vi "Autonomous Independent.vi"() -> ()   [LabVIEW 2014]
doc: "This VI is called when autonomous begins, and will automatically be terminated when autonomous ends. You can carry out timed or sensor driven robot movement independently without needing to return to the caller."
uses:
  <vilib>/Rock Robotics/WPI/SafetyOutput/WPI_SafetyOutputConfigMenu.ctl
  <vilib>/Rock Robotics/WPI/Joystick/WPI_JoystickGetSetRefNum.vi
  AutoVar.vi
  <vilib>/Rock Robotics/WPI/RobotDrive/WPI_RobotDriveGetSetRefNum.vi
  Global 2.vi
  <vilib>/Rock Robotics/WPI/RobotDrive/WPI_RobotDriveArcadeDrive_Standard(NoSaturation).vi
panel:
  out "Current Movement, for debugging":T1 {"Y Joystick Value" scale=1.0..-1.0; "X Joystick Value" scale=-1.0..1.0}
  in  "Array of robot movements":T2(array[cluster]) {"Y Joystick Value" scale=1.0..-1.0; "X Joystick Value" scale=-1.0..1.0}
  # "Be sure to right-click and choose Data Operations>>Make Current Value default if you want to save the array values with the VI"
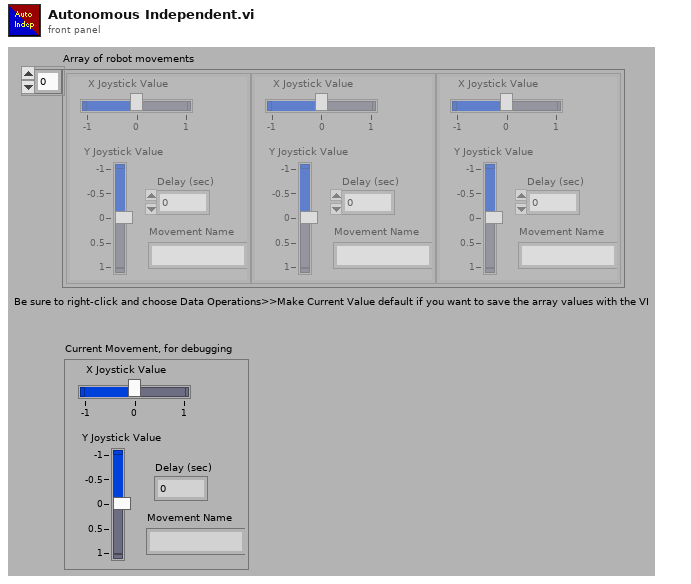
[diagram p1: front panel]
types:
  T1 = cluster{"X Joystick Value":dbl, "Y Joystick Value":dbl, "Delay (sec)":dbl, "Movement Name":string}
  T2 = cluster{"X Joystick Value":dbl, "Y Joystick Value":dbl, "Delay (sec)":dbl, "Movement Name":string}[]
  T3 = typedef "WPI_SafetyOutputConfigMenu.ctl" = enum16{"Enable", "Disable"}
  T4 = typedef "WPI_MotorControlDeviceRef.ctl" = cluster{"DeviceStatus":errorcluster, "Type":T5, "PWM":cluster{"Controller":T6, "PWM Channel":T7, "DeadBand":T8}, "CAN":cluster{"Device Number":u8, "Control Mode":T9, "Semaphore":T10, "Max Vout":dbl, "TalonSRX Control Mode":T11}, "Invert":bool, "TransformRef":T12, "InvTransformRef":T12}
  T5 = typedef "WPI_MotorControlType.ctl" = enum16{"PWM", "CAN", "CANTalonSRX"}
  T6 = typedef "FPGA_TypedefDigitalModule.ctl" = enum16{"Controller 1"}
  T7 = typedef "FPGA_DIOPWMChannel.ctl" = enum8{"PWM 0", "PWM 1", "PWM 2", "PWM 3", "PWM 4", "PWM 5", "PWM 6", "PWM 7", "PWM 8", "PWM 9", "PWM MXP 0", "PWM MXP 1", "PWM MXP 2", "PWM MXP 3", "PWM MXP 4", "PWM MXP 5", "PWM MXP 6", "PWM MXP 7", "PWM MXP 8", "PWM MXP 9", "Invalid"}
  T8 = typedef "WPI_PWMDeadband.ctl" = cluster{"Name":string, "maxPositivePwm":i32, "minPositivePwm":i32, "centerPwm":i32, "maxNegativePwm":i32, "minNegativePwm":i32, "angularRange":u16}
  T9 = typedef "WPI_CANJaguar_ControlMode.ctl" = enum8{"Percent VBus", "Current", "Speed", "Position", "Voltage"}
  T10 = typedef "Semaphore RefNum" = refnum<k1>
  T11 = typedef "WPI_CANTalonSRX_APIControlMode.ctl" = enum8{"Percent VBus", "Speed", "Position", "Slave", "Unchanged / Invalid"}
  T12 = typedef "WPI_PWMTransform_ConPane.ctl" = refnum<vi>
  T13 = typedef "WPI_RobotDriveDevRef.ctl" = cluster{"DevStatus":errorcluster, "Motors[]":T4[], "Square Inputs":bool, "Max Output":dbl}
  T14 = typedef "WPI_JoystickDevRef.ctl" = cluster{"Device":T15}
  T15 = typedef "WPI_JoystickDeviceEnum.ctl" = enum16{"USB 0", "USB 1", "USB 2", "USB 3", "USB 4", "USB 5"}
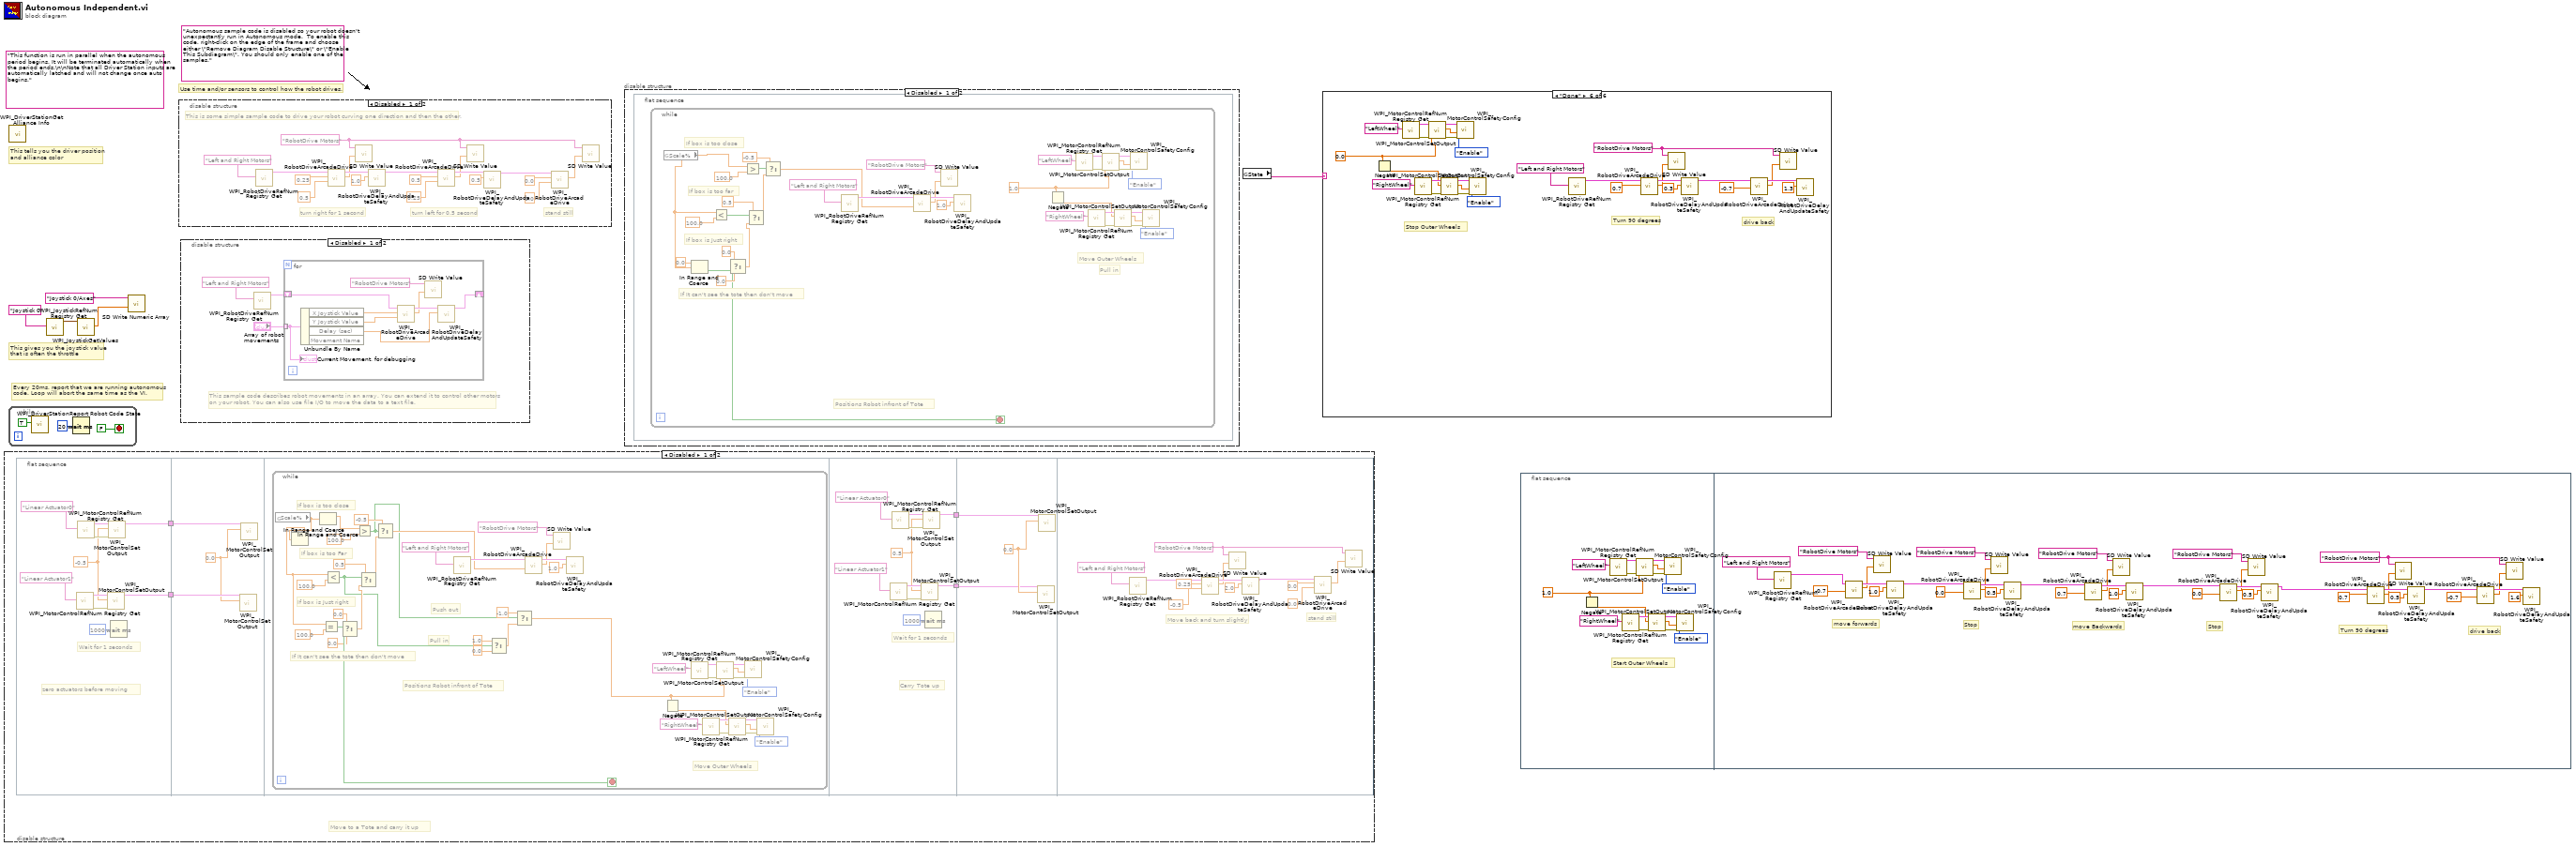
[diagram p0: block diagram]
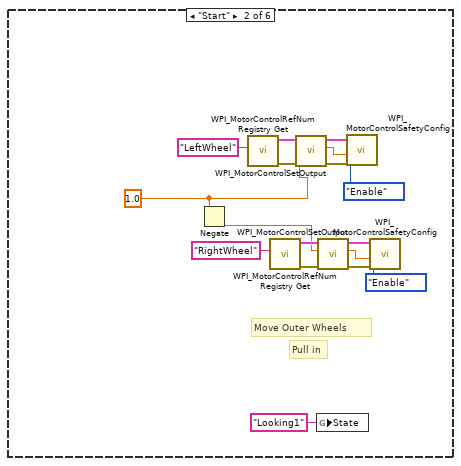
[diagram p4: hidden frame]
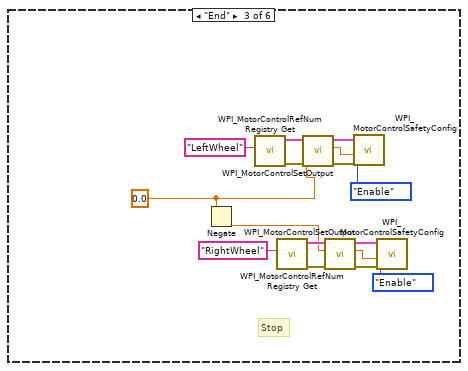
[diagram p5: hidden frame]
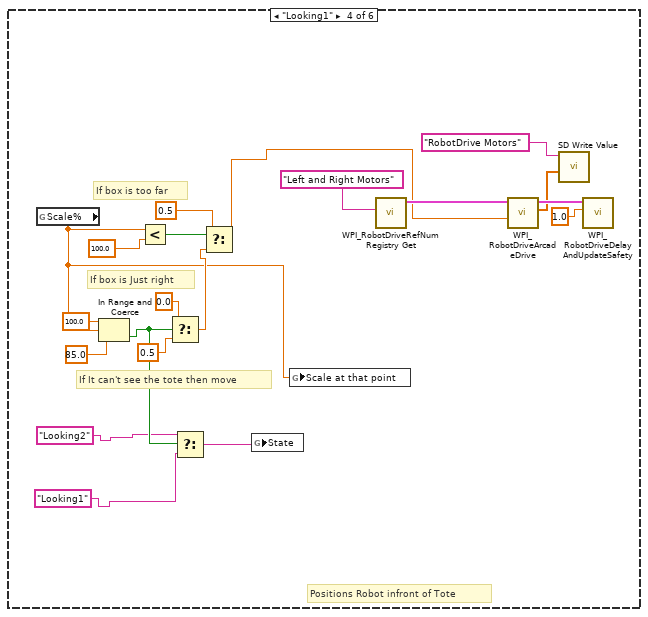
[diagram p6: hidden frame]
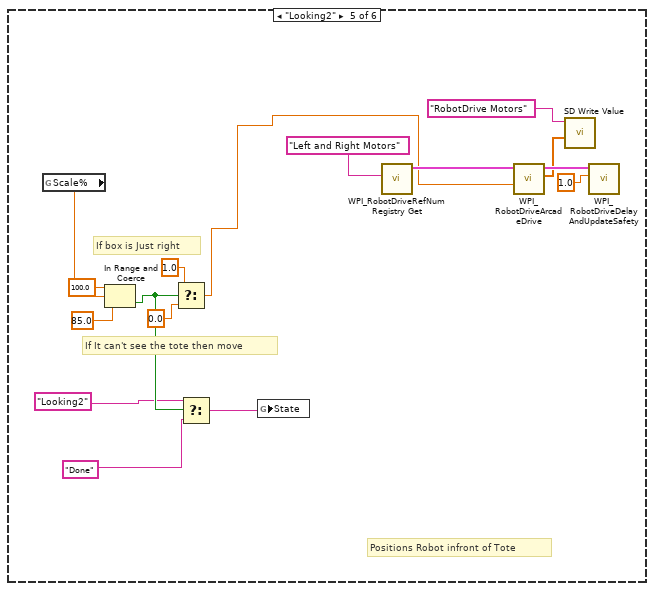
[diagram p7: hidden frame]
diagram:
  (unwired) "Autonomous sample code is disabled so your robot doesn't unexpectantly run in Autonomous mode.  To enable this code, right-click on the edge of the frame and choose either \"Remove Diagram Disable Structure\" or \"Enable This Subdiagram\". You should only enable one of the samples."
  (unwired) "This function is run in parallel when the autonomous period begins. It will be terminated automatically when the period ends.\n\nNote that all Driver Station inputs are automatically latched and will not change once auto begins."
  # "Every 20ms, report that we are running autonomous\ncode. Loop will abort the same time as the VI."
  # "This gives you the joystick value\nthat is often the throttle"
  # "Use time and/or sensors to control how the robot drives."
  # "This tells you the driver position\nand alliance color"
  n1 = disable-structure shown="Disabled" {
    frame Disabled {
      # "Move to a Tote and carry it up"
      n2 = flat-sequence {
        tunnel: [w11] -> w9
        tunnel: [w10] -> w8
        tunnel: w9 -> [w22]
        tunnel: w8 -> [w21]
        tunnel: [w66] -> w7
        tunnel: [w65] -> w6
        tunnel: w7 -> [w76]
        tunnel: w6 -> [w75]
        frame #0 {
          w13 = -0.5 ("Output")
          # "zero actuators before moving"
          # "Wait for 1 seconds"
          n3 = call <vilib>:"WPI_MotorControlRefNum Registry Get.vi"("refnum name"="Linear Actuator1") -> ("error out"=w16:errorcluster, "MotorControlDevRef"=w15:T4)  [unwired: 9 in]
          n4 = call <vilib>:"WPI_MotorControlRefNum Registry Get.vi"("refnum name"="Linear Actuator0") -> ("error out"=w19:errorcluster, "MotorControlDevRef"=w18:T4)  [unwired: 9 in]
          n5 = call <vilib>:"WPI_MotorControlSetOutput.vi"("error in (no error)"=w16, "Output"=w13, "MotorControlDevRef"=w15) -> ("MotorControlDevRef"=w10:T4)  [unwired: 6 in, 2 out]
          n6 = call <vilib>:"WPI_MotorControlSetOutput.vi"("error in (no error)"=w19, "Output"=w13, "MotorControlDevRef"=w18) -> ("MotorControlDevRef"=w11:T4)  [unwired: 6 in, 2 out]
          n7 = Wait (ms)(milliseconds to wait=u32 1000) -> ()  [unwired: 1 out]
        }
        frame #1 {
          w20 = 0.0 ("Output")
          n8 = call <vilib>:"WPI_MotorControlSetOutput.vi"("Output"=w20, "MotorControlDevRef"=w21) -> ()  [unwired: 7 in, 3 out]
          n9 = call <vilib>:"WPI_MotorControlSetOutput.vi"("Output"=w20, "MotorControlDevRef"=w22) -> ()  [unwired: 7 in, 3 out]
        }
        frame #2 {
          n10 = while {
            stop <- w49 stop-if-true
            # "Move Outer Wheels"
            # "Pull in"
            # "Push out"
            # "If It can't see the tote then don't move"
            # "Positions Robot infront of Tote"
            # "If box is Just right"
            # "If box is too Far"
            # "If box is too close"
            n11 = global read "Global 2.vi" "Scale%"() -> (w24:dbl)
            n12 = In Range and Coerce(x=w24) -> (coerced(x)=w23:dbl)  [unwired: 2 in, 1 out]
            n13 = In Range and Coerce(x=w24) -> (coerced(x)=w25:dbl)  [unwired: 2 in, 1 out]
            n14 = Equal?(x=w23, y=100.0) -> (x = y?=w49:bool)
            n15 = Less?(x=w23, y=100.0) -> (x < y?=w28:bool)
            n16 = Select(t=0.0, s=w49, f=0.0) -> (s? t:f=w57:dbl)
            n17 = Greater?(x=w25, y=100.0) -> (0:w33:bool)
            n18 = Select(t=0.5, s=w28, f=w57) -> (s? t:f=w60:dbl)
            n19 = Select(t=-0.5, s=w33, f=w60) -> (s? t:f=w50:dbl)
            n20 = call <vilib>:"WPI_RobotDriveRefNum Registry Get.vi"("refnum name"="Left and Right Motors") -> ("RobotDriveDevRef"=w53:T13)  [unwired: 1 in, 9 out]
            n21 = Select(t=1.0, s=w28, f=0.0) -> (s? t:f=w29:dbl)
            n22 = Select(t=-1.0, s=w33, f=w29) -> (s? t:f=w31:dbl)
            n23 = call-poly <vilib>:"WPI_RobotDriveArcadeDrive.vi"("Y axis value"=w50, "RobotDriveDevRef"=w53) -> ("Motor Values"=w52:dbl[], "RobotDriveDevRef"=w56:T13)  [unwired: 2 in, 6 out]
            n24 = call-poly <vilib>:"SD Write Value.vi"("Numeric Array"=w52, "Name"="RobotDrive Motors") -> ()  [unwired: 8 in, 2 out]
            n25 = call <vilib>:"WPI_RobotDriveDelayAndUpdateSafety.vi"("Delay (s)"=1.0, "RobotDriveDevRef"=w56) -> ()  [unwired: 8 in, 2 out]
            n26 = Negate(x=w31) -> (-x=w30:dbl)
            n27 = call <vilib>:"WPI_MotorControlRefNum Registry Get.vi"("refnum name"="LeftWheel") -> ("error out"=w47:errorcluster, "MotorControlDevRef"=w46:T4)  [unwired: 9 in]
            n28 = call <vilib>:"WPI_MotorControlRefNum Registry Get.vi"("refnum name"="RightWheel") -> ("error out"=w45:errorcluster, "MotorControlDevRef"=w44:T4)  [unwired: 9 in]
            n29 = call <vilib>:"WPI_MotorControlSetOutput.vi"("error in (no error)"=w47, "Output"=w31, "MotorControlDevRef"=w46) -> ("error out"=w41:errorcluster, "Motor Output"=w40:dbl, "MotorControlDevRef"=w39:T4)  [unwired: 6 in]
            n30 = call <vilib>:"WPI_MotorControlSetOutput.vi"("error in (no error)"=w45, "Output"=w30, "MotorControlDevRef"=w44) -> ("error out"=w38:errorcluster, "Motor Output"=w37:dbl, "MotorControlDevRef"=w36:T4)  [unwired: 6 in]
            n31 = call <vilib>:"WPI_MotorControlSafetyConfig.vi"("error in (no error)"=w41, "timeout (s)"=w40, "mode"=WPI_SafetyOutputConfigMenu."Enable", "MotorControlDevRef"=w39) -> ()  [unwired: 6 in, 2 out]
            n32 = call <vilib>:"WPI_MotorControlSafetyConfig.vi"("error in (no error)"=w38, "timeout (s)"=w37, "mode"=WPI_SafetyOutputConfigMenu."Enable", "MotorControlDevRef"=w36) -> ()  [unwired: 6 in, 2 out]
          }
        }
        frame #3 {
          w68 = 0.5 ("Output")
          # "Carry Tote up"
          # "Wait for 1 seconds"
          n33 = call <vilib>:"WPI_MotorControlRefNum Registry Get.vi"("refnum name"="Linear Actuator1") -> ("error out"=w71:errorcluster, "MotorControlDevRef"=w70:T4)  [unwired: 9 in]
          n34 = call <vilib>:"WPI_MotorControlRefNum Registry Get.vi"("refnum name"="Linear Actuator0") -> ("error out"=w74:errorcluster, "MotorControlDevRef"=w73:T4)  [unwired: 9 in]
          n35 = call <vilib>:"WPI_MotorControlSetOutput.vi"("error in (no error)"=w71, "Output"=w68, "MotorControlDevRef"=w70) -> ("MotorControlDevRef"=w65:T4)  [unwired: 6 in, 2 out]
          n36 = call <vilib>:"WPI_MotorControlSetOutput.vi"("error in (no error)"=w74, "Output"=w68, "MotorControlDevRef"=w73) -> ("MotorControlDevRef"=w66:T4)  [unwired: 6 in, 2 out]
          n37 = Wait (ms)(milliseconds to wait=u32 1000) -> ()  [unwired: 1 out]
        }
        frame #4 {
          w77 = 0.0 ("Output")
          n38 = call <vilib>:"WPI_MotorControlSetOutput.vi"("Output"=w77, "MotorControlDevRef"=w75) -> ()  [unwired: 7 in, 3 out]
          n39 = call <vilib>:"WPI_MotorControlSetOutput.vi"("Output"=w77, "MotorControlDevRef"=w76) -> ()  [unwired: 7 in, 3 out]
        }
        frame #5 {
          w78 = "RobotDrive Motors" ("Name")
          # "stand still"
          # "Move back and turn slightly"
          n40 = call <vilib>:"WPI_RobotDriveRefNum Registry Get.vi"("refnum name"="Left and Right Motors") -> ("RobotDriveDevRef"=w85:T13)  [unwired: 1 in, 9 out]
          n41 = call-poly <vilib>:"WPI_RobotDriveArcadeDrive.vi"("Y axis value"=-0.5 ("X axis value"), "X axis value"=0.25, "RobotDriveDevRef"=w85) -> ("Motor Values"=w84:dbl[], "RobotDriveDevRef"=w88:T13)  [unwired: 1 in, 6 out]
          n42 = call-poly <vilib>:"SD Write Value.vi"("Numeric Array"=w84, "Name"=w78) -> ()  [unwired: 8 in, 2 out]
          n43 = call <vilib>:"WPI_RobotDriveDelayAndUpdateSafety.vi"("Delay (s)"=2.0, "RobotDriveDevRef"=w88) -> ("RobotDriveDevRef 2"=w79:T13)  [unwired: 8 in, 1 out]
          n44 = call-poly <vilib>:"WPI_RobotDriveArcadeDrive.vi"("Y axis value"=0.0 ("X axis value"), "X axis value"=0.0, "RobotDriveDevRef"=w79) -> ("Motor Values"=w80:dbl[])  [unwired: 1 in, 7 out]
          n45 = call-poly <vilib>:"SD Write Value.vi"("Numeric Array"=w80, "Name"=w78) -> ()  [unwired: 8 in, 2 out]
        }
      }
    }
    frame Enabled {
    }
  }
  n46 = while {
    stop <- FALSE stop-if-true
    n47 = call <vilib>:"WPI_DriverStationReport Robot Code State.vi"("Autonomous"=TRUE) -> ()  [unwired: 10 in, 1 out]
    n48 = Wait (ms)(milliseconds to wait=u32 20) -> ()  [unwired: 1 out]
  }
  n49 = call <vilib>:"WPI_DriverStationGet Alliance Info.vi"() -> ()  [unwired: 12 out]
  n50 = call <vilib>:"WPI_JoystickRefNum Registry Get.vi"("refnum name"="Joystick 0") -> ("JoystickDevRef"=w4:T14)  [unwired: 1 in, 9 out]
  n51 = call <vilib>:"WPI_JoystickGetValues.vi"("JoystickDevRef"=w4) -> ("Axes"=w2:dbl[])  [unwired: 6 in, 4 out]
  n52 = call <vilib>:"SD Write Numeric Array.vi"("Numeric Array"=w2, "Name"="Joystick 0/Axes") -> ()  [unwired: 8 in, 2 out]
  n53 = disable-structure shown="Disabled" {
    frame Disabled {
      w93 = "RobotDrive Motors" ("Name")
      # "This is some simple sample code to drive your robot curving one direction and then the other."
      # "stand still"
      # "turn left for 0.5 second"
      # "turn right for 1 second"
      n54 = call <vilib>:"WPI_RobotDriveRefNum Registry Get.vi"("refnum name"="Left and Right Motors") -> ("RobotDriveDevRef"=w97:T13)  [unwired: 1 in, 9 out]
      n55 = call-poly <vilib>:"WPI_RobotDriveArcadeDrive.vi"("Y axis value"=0.5 ("X axis value"), "X axis value"=0.25, "RobotDriveDevRef"=w97) -> ("Motor Values"=w96:dbl[], "RobotDriveDevRef"=w104:T13)  [unwired: 1 in, 6 out]
      n56 = call-poly <vilib>:"SD Write Value.vi"("Numeric Array"=w96, "Name"=w93) -> ()  [unwired: 8 in, 2 out]
      n57 = call <vilib>:"WPI_RobotDriveDelayAndUpdateSafety.vi"("Delay (s)"=1.0, "RobotDriveDevRef"=w104) -> ("RobotDriveDevRef 2"=w103:T13)  [unwired: 8 in, 1 out]
      n58 = call-poly <vilib>:"WPI_RobotDriveArcadeDrive.vi"("Y axis value"=0.25 ("X axis value"), "X axis value"=0.5, "RobotDriveDevRef"=w103) -> ("Motor Values"=w95:dbl[], "RobotDriveDevRef"=w102:T13)  [unwired: 1 in, 6 out]
      n59 = call-poly <vilib>:"SD Write Value.vi"("Numeric Array"=w95, "Name"=w93) -> ()  [unwired: 8 in, 2 out]
      n60 = call <vilib>:"WPI_RobotDriveDelayAndUpdateSafety.vi"("Delay (s)"=0.5, "RobotDriveDevRef"=w102) -> ("RobotDriveDevRef 2"=w101:T13)  [unwired: 8 in, 1 out]
      n61 = call-poly <vilib>:"WPI_RobotDriveArcadeDrive.vi"("Y axis value"=0.0 ("X axis value"), "X axis value"=0.0, "RobotDriveDevRef"=w101) -> ("Motor Values"=w94:dbl[])  [unwired: 1 in, 7 out]
      n62 = call-poly <vilib>:"SD Write Value.vi"("Numeric Array"=w94, "Name"=w93) -> ()  [unwired: 8 in, 2 out]
    }
    frame Enabled {
    }
  }
  n63 = disable-structure shown="Disabled" {
    frame Disabled {
      # "This sample code describes robot movements in an array. You can extend it to control other motors\non your robot. You can also use file I/O to move the data to a text file."
      n64 = call <vilib>:"WPI_RobotDriveRefNum Registry Get.vi"("refnum name"="Left and Right Motors") -> ("RobotDriveDevRef"=w112:T13)  [unwired: 1 in, 9 out]
      n65 = for {
        shift-right: [w120] -> _
        shift-left: w112 -> [w121]
        tunnel: "Array of robot movements" -> [w116] mode=indexing
        n66 = Unbundle By Name(w116) -> ("X Joystick Value"=w119:dbl, "Y Joystick Value"=w118:dbl, "Delay (sec)"=w117:dbl)  [unwired: 1 out]
        n67 = call-poly <vilib>:"WPI_RobotDriveArcadeDrive.vi"("Y axis value"=w118, "X axis value"=w119, "RobotDriveDevRef"=w121) -> ("Motor Values"=w114:dbl[], "RobotDriveDevRef"=w122:T13)  [unwired: 1 in, 6 out]
        n68 = call-poly <vilib>:"SD Write Value.vi"("Numeric Array"=w114, "Name"="RobotDrive Motors") -> ()  [unwired: 8 in, 2 out]
        n69 = call <vilib>:"WPI_RobotDriveDelayAndUpdateSafety.vi"("Delay (s)"=w117, "RobotDriveDevRef"=w122) -> ("RobotDriveDevRef 2"=w120:T13)  [unwired: 8 in, 1 out]
        "Current Movement, for debugging" <- w116
      }
    }
    frame Enabled {
    }
  }
  n70 = disable-structure shown="Disabled" {
    frame Disabled {
      n71 = flat-sequence {
        frame #0 {
          n72 = while {
            stop <- w126 stop-if-true
            w123 = 1.0 ("t")
            # "Move Outer Wheels"
            # "Pull in"
            # "If It can't see the tote then don't move"
            # "Positions Robot infront of Tote"
            # "If box is Just right"
            # "If box is too far"
            # "If box is too close"
            n73 = global read "Global 2.vi" "Scale%"() -> (w125:dbl)
            n74 = In Range and Coerce(upper limit=0.0, x=w125) -> (In Range?=w126:bool)  [unwired: 1 in, 1 out]
            n75 = Less?(x=w125, y=100.0) -> (x < y?=w127:bool)
            n76 = Select(t=0.0, s=w126, f=0.0) -> (s? t:f=w152:dbl)
            n77 = Greater?(x=w125, y=100.0) -> (0:w129:bool)
            n78 = Select(t=0.5, s=w127, f=w152) -> (s? t:f=w154:dbl)
            n79 = Select(t=-0.5, s=w129, f=w154) -> (s? t:f=w145:dbl)
            n80 = call <vilib>:"WPI_RobotDriveRefNum Registry Get.vi"("refnum name"="Left and Right Motors") -> ("RobotDriveDevRef"=w148:T13)  [unwired: 1 in, 9 out]
            n81 = call-poly <vilib>:"WPI_RobotDriveArcadeDrive.vi"("Y axis value"=w145, "RobotDriveDevRef"=w148) -> ("Motor Values"=w147:dbl[], "RobotDriveDevRef"=w151:T13)  [unwired: 2 in, 6 out]
            n82 = call-poly <vilib>:"SD Write Value.vi"("Numeric Array"=w147, "Name"="RobotDrive Motors") -> ()  [unwired: 8 in, 2 out]
            n83 = call <vilib>:"WPI_RobotDriveDelayAndUpdateSafety.vi"("Delay (s)"=1.0, "RobotDriveDevRef"=w151) -> ()  [unwired: 8 in, 2 out]
            n84 = Negate(x=w123) -> (-x=w128:dbl)
            n85 = call <vilib>:"WPI_MotorControlRefNum Registry Get.vi"("refnum name"="LeftWheel") -> ("error out"=w143:errorcluster, "MotorControlDevRef"=w142:T4)  [unwired: 9 in]
            n86 = call <vilib>:"WPI_MotorControlRefNum Registry Get.vi"("refnum name"="RightWheel") -> ("error out"=w141:errorcluster, "MotorControlDevRef"=w140:T4)  [unwired: 9 in]
            n87 = call <vilib>:"WPI_MotorControlSetOutput.vi"("error in (no error)"=w143, "Output"=w123, "MotorControlDevRef"=w142) -> ("error out"=w137:errorcluster, "Motor Output"=w136:dbl, "MotorControlDevRef"=w135:T4)  [unwired: 6 in]
            n88 = call <vilib>:"WPI_MotorControlSetOutput.vi"("error in (no error)"=w141, "Output"=w128, "MotorControlDevRef"=w140) -> ("error out"=w134:errorcluster, "Motor Output"=w133:dbl, "MotorControlDevRef"=w132:T4)  [unwired: 6 in]
            n89 = call <vilib>:"WPI_MotorControlSafetyConfig.vi"("error in (no error)"=w137, "timeout (s)"=w136, "mode"=WPI_SafetyOutputConfigMenu."Enable", "MotorControlDevRef"=w135) -> ()  [unwired: 6 in, 2 out]
            n90 = call <vilib>:"WPI_MotorControlSafetyConfig.vi"("error in (no error)"=w134, "timeout (s)"=w133, "mode"=WPI_SafetyOutputConfigMenu."Enable", "MotorControlDevRef"=w132) -> ()  [unwired: 6 in, 2 out]
          }
        }
      }
    }
    frame Enabled {
    }
  }
  n91 = global read "AutoVar.vi" "State"() -> (w1:string)
  n92 = case shown="\"Done\"" w1 {
    frame "False", Default {
    }
    frame "Start" {
      w160 = 1.0 ("t")
      # "Move Outer Wheels"
      # "Pull in"
      n93 = Negate(x=w160) -> (-x=w161:dbl)
      n94 = call <vilib>:"WPI_MotorControlRefNum Registry Get.vi"("refnum name"="LeftWheel") -> ("error out"=w175:errorcluster, "MotorControlDevRef"=w174:T4)  [unwired: 9 in]
      n95 = call <vilib>:"WPI_MotorControlRefNum Registry Get.vi"("refnum name"="RightWheel") -> ("error out"=w173:errorcluster, "MotorControlDevRef"=w172:T4)  [unwired: 9 in]
      n96 = call <vilib>:"WPI_MotorControlSetOutput.vi"("error in (no error)"=w175, "Output"=w160, "MotorControlDevRef"=w174) -> ("error out"=w169:errorcluster, "Motor Output"=w168:dbl, "MotorControlDevRef"=w167:T4)  [unwired: 6 in]
      n97 = global write "AutoVar.vi" "State"("Looking1" ("State")) -> ()
      n98 = call <vilib>:"WPI_MotorControlSetOutput.vi"("error in (no error)"=w173, "Output"=w161, "MotorControlDevRef"=w172) -> ("error out"=w166:errorcluster, "Motor Output"=w165:dbl, "MotorControlDevRef"=w164:T4)  [unwired: 6 in]
      n99 = call <vilib>:"WPI_MotorControlSafetyConfig.vi"("error in (no error)"=w169, "timeout (s)"=w168, "mode"=WPI_SafetyOutputConfigMenu."Enable", "MotorControlDevRef"=w167) -> ()  [unwired: 6 in, 2 out]
      n100 = call <vilib>:"WPI_MotorControlSafetyConfig.vi"("error in (no error)"=w166, "timeout (s)"=w165, "mode"=WPI_SafetyOutputConfigMenu."Enable", "MotorControlDevRef"=w164) -> ()  [unwired: 6 in, 2 out]
    }
    frame "End" {
      w176 = 0.0 ("t")
      # "Stop"
      n101 = Negate(x=w176) -> (-x=w177:dbl)
      n102 = call <vilib>:"WPI_MotorControlRefNum Registry Get.vi"("refnum name"="LeftWheel") -> ("error out"=w191:errorcluster, "MotorControlDevRef"=w190:T4)  [unwired: 9 in]
      n103 = call <vilib>:"WPI_MotorControlRefNum Registry Get.vi"("refnum name"="RightWheel") -> ("error out"=w189:errorcluster, "MotorControlDevRef"=w188:T4)  [unwired: 9 in]
      n104 = call <vilib>:"WPI_MotorControlSetOutput.vi"("error in (no error)"=w191, "Output"=w176, "MotorControlDevRef"=w190) -> ("error out"=w185:errorcluster, "Motor Output"=w184:dbl, "MotorControlDevRef"=w183:T4)  [unwired: 6 in]
      n105 = call <vilib>:"WPI_MotorControlSetOutput.vi"("error in (no error)"=w189, "Output"=w177, "MotorControlDevRef"=w188) -> ("error out"=w182:errorcluster, "Motor Output"=w181:dbl, "MotorControlDevRef"=w180:T4)  [unwired: 6 in]
      n106 = call <vilib>:"WPI_MotorControlSafetyConfig.vi"("error in (no error)"=w185, "timeout (s)"=w184, "mode"=WPI_SafetyOutputConfigMenu."Enable", "MotorControlDevRef"=w183) -> ()  [unwired: 6 in, 2 out]
      n107 = call <vilib>:"WPI_MotorControlSafetyConfig.vi"("error in (no error)"=w182, "timeout (s)"=w181, "mode"=WPI_SafetyOutputConfigMenu."Enable", "MotorControlDevRef"=w180) -> ()  [unwired: 6 in, 2 out]
    }
    frame "Looking1" {
      # "If It can't see the tote then move"
      # "Positions Robot infront of Tote"
      # "If box is Just right"
      # "If box is too far"
      n108 = global read "Global 2.vi" "Scale%"() -> (w194:dbl)
      n109 = In Range and Coerce(upper limit=100.0, x=w194, lower limit=85.0) -> (In Range?=w196:bool)  [unwired: 1 out]
      n110 = Less?(x=w194, y=100.0) -> (x < y?=w201:bool)
      n111 = Select(t=0.0, s=w196, f=0.5) -> (s? t:f=w208:dbl)
      n112 = Select(t="Looking2", s=w196, f="Looking1" ("t")) -> (s? t:f=w195:string)
      n113 = Select(t=0.5, s=w201, f=w208) -> (s? t:f=w198:dbl)
      n114 = global write "AutoVar.vi" "State"(w195) -> ()
      n115 = global write "AutoVar.vi" "Scale at that point"(w194) -> ()
      n116 = call <vilib>:"WPI_RobotDriveRefNum Registry Get.vi"("refnum name"="Left and Right Motors") -> ("RobotDriveDevRef"=w204:T13)  [unwired: 1 in, 9 out]
      n117 = call-poly <vilib>:"WPI_RobotDriveArcadeDrive.vi"("Y axis value"=w198, "RobotDriveDevRef"=w204) -> ("Motor Values"=w203:dbl[], "RobotDriveDevRef"=w207:T13)  [unwired: 2 in, 6 out]
      n118 = call-poly <vilib>:"SD Write Value.vi"("Numeric Array"=w203, "Name"="RobotDrive Motors") -> ()  [unwired: 8 in, 2 out]
      n119 = call <vilib>:"WPI_RobotDriveDelayAndUpdateSafety.vi"("Delay (s)"=1.0, "RobotDriveDevRef"=w207) -> ()  [unwired: 8 in, 2 out]
    }
    frame "Looking2" {
      # "If It can't see the tote then move"
      # "Positions Robot infront of Tote"
      # "If box is Just right"
      n120 = global read "Global 2.vi" "Scale%"() -> (w220:dbl)
      n121 = In Range and Coerce(upper limit=100.0, x=w220, lower limit=85.0) -> (In Range?=w216:bool)  [unwired: 1 out]
      n122 = Select(t=1.0, s=w216, f=0.0) -> (s? t:f=w214:dbl)
      n123 = Select(t="Looking2", s=w216, f="Done" ("t")) -> (s? t:f=w215:string)
      n124 = global write "AutoVar.vi" "State"(w215) -> ()
      n125 = call <vilib>:"WPI_RobotDriveRefNum Registry Get.vi"("refnum name"="Left and Right Motors") -> ("RobotDriveDevRef"=w223:T13)  [unwired: 1 in, 9 out]
      n126 = call-poly <vilib>:"WPI_RobotDriveArcadeDrive.vi"("Y axis value"=w214, "RobotDriveDevRef"=w223) -> ("Motor Values"=w222:dbl[], "RobotDriveDevRef"=w226:T13)  [unwired: 2 in, 6 out]
      n127 = call-poly <vilib>:"SD Write Value.vi"("Numeric Array"=w222, "Name"="RobotDrive Motors") -> ()  [unwired: 8 in, 2 out]
      n128 = call <vilib>:"WPI_RobotDriveDelayAndUpdateSafety.vi"("Delay (s)"=1.0, "RobotDriveDevRef"=w226) -> ()  [unwired: 8 in, 2 out]
    }
    frame "Done" {
      w229 = "RobotDrive Motors" ("Name")
      w240 = 0.0 ("t")
      # "drive back"
      # "Turn 90 degrees"
      # "Stop Outer Wheels"
      n129 = Negate(x=w240) -> (-x=w241:dbl)
      n130 = call <vilib>:"WPI_MotorControlRefNum Registry Get.vi"("refnum name"="LeftWheel") -> ("error out"=w255:errorcluster, "MotorControlDevRef"=w254:T4)  [unwired: 9 in]
      n131 = call <vilib>:"WPI_MotorControlRefNum Registry Get.vi"("refnum name"="RightWheel") -> ("error out"=w253:errorcluster, "MotorControlDevRef"=w252:T4)  [unwired: 9 in]
      n132 = call <vilib>:"WPI_MotorControlSetOutput.vi"("error in (no error)"=w255, "Output"=w240, "MotorControlDevRef"=w254) -> ("error out"=w249:errorcluster, "Motor Output"=w248:dbl, "MotorControlDevRef"=w247:T4)  [unwired: 6 in]
      n133 = call <vilib>:"WPI_MotorControlSetOutput.vi"("error in (no error)"=w253, "Output"=w241, "MotorControlDevRef"=w252) -> ("error out"=w246:errorcluster, "Motor Output"=w245:dbl, "MotorControlDevRef"=w244:T4)  [unwired: 6 in]
      n134 = call <vilib>:"WPI_MotorControlSafetyConfig.vi"("error in (no error)"=w249, "timeout (s)"=w248, "mode"=WPI_SafetyOutputConfigMenu."Enable", "MotorControlDevRef"=w247) -> ()  [unwired: 6 in, 2 out]
      n135 = call <vilib>:"WPI_MotorControlSafetyConfig.vi"("error in (no error)"=w246, "timeout (s)"=w245, "mode"=WPI_SafetyOutputConfigMenu."Enable", "MotorControlDevRef"=w244) -> ()  [unwired: 6 in, 2 out]
      n136 = call <vilib>:"WPI_RobotDriveRefNum Registry Get.vi"("refnum name"="Left and Right Motors") -> ("RobotDriveDevRef"=w232:T13)  [unwired: 1 in, 9 out]
      n137 = call-poly <vilib>:"WPI_RobotDriveArcadeDrive.vi"("X axis value"=0.7, "RobotDriveDevRef"=w232) -> ("Motor Values"=w231:dbl[], "RobotDriveDevRef"=w238:T13)  [unwired: 2 in, 6 out]
      n138 = call-poly <vilib>:"SD Write Value.vi"("Numeric Array"=w231, "Name"=w229) -> ()  [unwired: 8 in, 2 out]
      n139 = call <vilib>:"WPI_RobotDriveDelayAndUpdateSafety.vi"("Delay (s)"=0.3, "RobotDriveDevRef"=w238) -> ("RobotDriveDevRef 2"=w237:T13)  [unwired: 8 in, 1 out]
      n140 = call-poly <vilib>:"WPI_RobotDriveArcadeDrive.vi"("Y axis value"=-0.7 ("X axis value"), "RobotDriveDevRef"=w237) -> ("Motor Values"=w230:dbl[], "RobotDriveDevRef"=w236:T13)  [unwired: 2 in, 6 out]
      n141 = call-poly <vilib>:"SD Write Value.vi"("Numeric Array"=w230, "Name"=w229) -> ()  [unwired: 8 in, 2 out]
      n142 = call <vilib>:"WPI_RobotDriveDelayAndUpdateSafety.vi"("Delay (s)"=1.3, "RobotDriveDevRef"=w236) -> ()  [unwired: 8 in, 2 out]
    }
  }
  n143 = flat-sequence {
    frame #0 {
      w256 = 1.0 ("t")
      # "Start Outer Wheels"
      n144 = Negate(x=w256) -> (-x=w257:dbl)
      n145 = call <vilib>:"WPI_MotorControlRefNum Registry Get.vi"("refnum name"="LeftWheel") -> ("error out"=w271:errorcluster, "MotorControlDevRef"=w270:T4)  [unwired: 9 in]
      n146 = call <vilib>:"WPI_MotorControlRefNum Registry Get.vi"("refnum name"="RightWheel") -> ("error out"=w269:errorcluster, "MotorControlDevRef"=w268:T4)  [unwired: 9 in]
      n147 = call <vilib>:"WPI_MotorControlSetOutput.vi"("error in (no error)"=w271, "Output"=w256, "MotorControlDevRef"=w270) -> ("error out"=w265:errorcluster, "Motor Output"=w264:dbl, "MotorControlDevRef"=w263:T4)  [unwired: 6 in]
      n148 = call <vilib>:"WPI_MotorControlSetOutput.vi"("error in (no error)"=w269, "Output"=w257, "MotorControlDevRef"=w268) -> ("error out"=w262:errorcluster, "Motor Output"=w261:dbl, "MotorControlDevRef"=w260:T4)  [unwired: 6 in]
      n149 = call <vilib>:"WPI_MotorControlSafetyConfig.vi"("error in (no error)"=w265, "timeout (s)"=w264, "mode"=WPI_SafetyOutputConfigMenu."Enable", "MotorControlDevRef"=w263) -> ()  [unwired: 6 in, 2 out]
      n150 = call <vilib>:"WPI_MotorControlSafetyConfig.vi"("error in (no error)"=w262, "timeout (s)"=w261, "mode"=WPI_SafetyOutputConfigMenu."Enable", "MotorControlDevRef"=w260) -> ()  [unwired: 6 in, 2 out]
    }
    frame #1 {
      w298 = "RobotDrive Motors" ("Name")
      # "Stop"
      # "move Backwards"
      # "Stop"
      # "move forwards"
      # "drive back"
      # "Turn 90 degrees"
      n151 = call <vilib>:"WPI_RobotDriveRefNum Registry Get.vi"("refnum name"="Left and Right Motors") -> ("RobotDriveDevRef"=w293:T13)  [unwired: 1 in, 9 out]
      n152 = call-poly <vilib>:"WPI_RobotDriveArcadeDrive.vi"("Y axis value"=-0.7 ("X axis value"), "RobotDriveDevRef"=w293) -> ("Motor Values"=w295:dbl[], "RobotDriveDevRef"=w297:T13)  [unwired: 2 in, 6 out]
      n153 = call-poly <vilib>:"SD Write Value.vi"("Numeric Array"=w295, "Name"="RobotDrive Motors") -> ()  [unwired: 8 in, 2 out]
      n154 = call <vilib>:"WPI_RobotDriveDelayAndUpdateSafety.vi"("Delay (s)"=1.0, "RobotDriveDevRef"=w297) -> ("RobotDriveDevRef 2"=w285:T13)  [unwired: 8 in, 1 out]
      n155 = call-poly <vilib>:"WPI_RobotDriveArcadeDrive.vi"("Y axis value"=0.0 ("X axis value"), "RobotDriveDevRef"=w285) -> ("Motor Values"=w288:dbl[], "RobotDriveDevRef"=w290:T13)  [unwired: 2 in, 6 out]
      n156 = call-poly <vilib>:"SD Write Value.vi"("Numeric Array"=w288, "Name"="RobotDrive Motors") -> ()  [unwired: 8 in, 2 out]
      n157 = call <vilib>:"WPI_RobotDriveDelayAndUpdateSafety.vi"("Delay (s)"=0.5, "RobotDriveDevRef"=w290) -> ("RobotDriveDevRef 2"=w279:T13)  [unwired: 8 in, 1 out]
      n158 = call-poly <vilib>:"WPI_RobotDriveArcadeDrive.vi"("Y axis value"=0.7 ("X axis value"), "RobotDriveDevRef"=w279) -> ("Motor Values"=w282:dbl[], "RobotDriveDevRef"=w284:T13)  [unwired: 2 in, 6 out]
      n159 = call-poly <vilib>:"SD Write Value.vi"("Numeric Array"=w282, "Name"="RobotDrive Motors") -> ()  [unwired: 8 in, 2 out]
      n160 = call <vilib>:"WPI_RobotDriveDelayAndUpdateSafety.vi"("Delay (s)"=1.0, "RobotDriveDevRef"=w284) -> ("RobotDriveDevRef 2"=w273:T13)  [unwired: 8 in, 1 out]
      n161 = call-poly <vilib>:"WPI_RobotDriveArcadeDrive.vi"("Y axis value"=0.0 ("X axis value"), "RobotDriveDevRef"=w273) -> ("Motor Values"=w276:dbl[], "RobotDriveDevRef"=w278:T13)  [unwired: 2 in, 6 out]
      n162 = call-poly <vilib>:"SD Write Value.vi"("Numeric Array"=w276, "Name"="RobotDrive Motors") -> ()  [unwired: 8 in, 2 out]
      n163 = call <vilib>:"WPI_RobotDriveDelayAndUpdateSafety.vi"("Delay (s)"=0.5, "RobotDriveDevRef"=w278) -> ("RobotDriveDevRef 2"=w272:T13)  [unwired: 8 in, 1 out]
      n164 = call-poly <vilib>:"WPI_RobotDriveArcadeDrive.vi"("X axis value"=0.7, "RobotDriveDevRef"=w272) -> ("Motor Values"=w300:dbl[], "RobotDriveDevRef"=w306:T13)  [unwired: 2 in, 6 out]
      n165 = call-poly <vilib>:"SD Write Value.vi"("Numeric Array"=w300, "Name"=w298) -> ()  [unwired: 8 in, 2 out]
      n166 = call <vilib>:"WPI_RobotDriveDelayAndUpdateSafety.vi"("Delay (s)"=0.5, "RobotDriveDevRef"=w306) -> ("RobotDriveDevRef 2"=w305:T13)  [unwired: 8 in, 1 out]
      n167 = call-poly <vilib>:"WPI_RobotDriveArcadeDrive.vi"("Y axis value"=-0.7 ("X axis value"), "RobotDriveDevRef"=w305) -> ("Motor Values"=w299:dbl[], "RobotDriveDevRef"=w304:T13)  [unwired: 2 in, 6 out]
      n168 = call-poly <vilib>:"SD Write Value.vi"("Numeric Array"=w299, "Name"=w298) -> ()  [unwired: 8 in, 2 out]
      n169 = call <vilib>:"WPI_RobotDriveDelayAndUpdateSafety.vi"("Delay (s)"=1.6, "RobotDriveDevRef"=w304) -> ()  [unwired: 8 in, 2 out]
    }
  }
